vi "Import data from S2DS- B Reader.vi"(8 "error in (no error)":errorcluster) -> (0 "error out":errorcluster, 2 "Data out":dbl[](array[numeric]), 3 "connection out":refnum<k13>)   [LabVIEW 2016]
doc: "Uses DataSocket to read array data. \n \nThe Writer, Server, and Reader can all be on the same computer or different computers. The Writer and Reader URLs should point to the computer where the DataSocket Server is."
uses:
  source/INST DRIVERS/DilutionFridge/MyTriton.lvlib
panel:
  out "VISA resource name out":refnum<visa-resource-name>
  out "B":dbl
  in  "error in (no error) 2":errorcluster
  in  "VISA resource name in":refnum<visa-resource-name>="TCPIP0::192.168.0.107::33576::SOCKET"
  out "error out 2":errorcluster
  # "Overview: Demonstrates the use of the DataSocket functions to read data from the DataSocket server of S2DS.\nRequirements: Windows\nInstructions:\n1. Ensure Simple 2D Sweep : Export data  is TRUE.\n2. Run the VI."
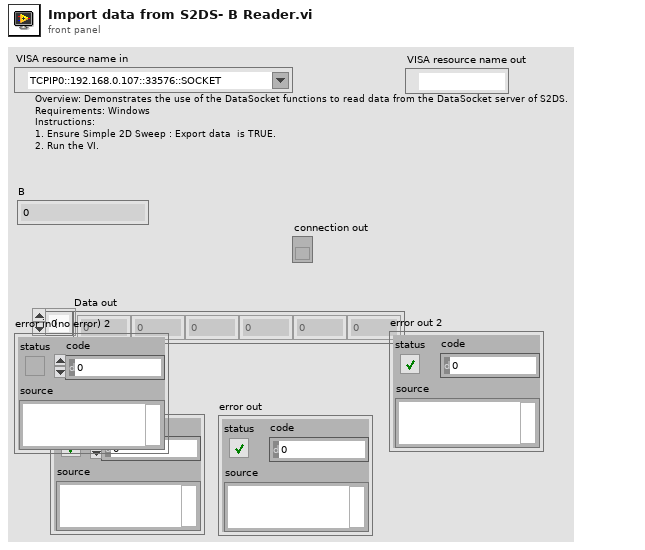
[diagram p1: front panel]
types:
  T1 = enum16{"Read", "Write", "ReadWrite", "BufferedRead", "BufferedReadWrite"}
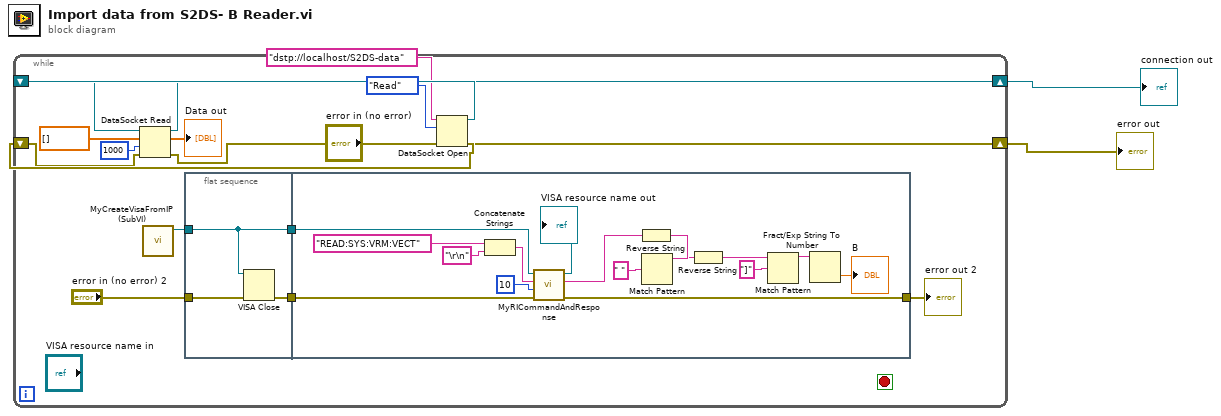
[diagram p0: block diagram]
diagram:
  n1 = DataSocket Open(8:"error in (no error)", 10:T1."Read" ("mode"), 11:"dstp://localhost/S2DS-data" ("Read Location")) -> (0:w4:errorcluster, 3:w6:refnum<k13>)  [unwired: 1 in]
  n2 = while {
    shift-right: [w13] -> w3
    shift-left: w6 -> [w15]
    shift-right: [w16] -> w7
    shift-left: w4 -> [w14]
    stop <- _ stop-if-true
    n3 = DataSocket Read(8:w14, 9:1000 ("ms timeout (10000)"), 10:dbl[] [], 11:w15) -> (0:w16:errorcluster, 2:→"Data out":dbl[], 3:w13:refnum<k13>)  [unwired: 5 out]
    n4 = call "MyCreateVisaFromIP (SubVI).vi"() -> ("VISA Refnum out"=w8:refnum<visa-resource-name>)  [unwired: 11 in]
    n5 = flat-sequence {
      tunnel: w8 -> [w20]
      tunnel: "error in (no error) 2" -> [w22]
      tunnel: [w21] -> w12
      tunnel: [w20] -> w11
      tunnel: w12 -> [w25]
      tunnel: w11 -> [w24]
      tunnel: [w23] -> w10
      frame #0 {
        n6 = VISA Close(VISA resource name=w20, error in (no error)=w22) -> (error out=w21:errorcluster)
      }
      frame #1 {
        n7 = Concatenate Strings("READ:SYS:VRM:VECT" ("Command"), "\r\n" ("string")) -> (w36:string)
        n8 = call "MyRICommandAndResponse.vi"("error in (no error)"=w25, "Min byte count"=u32 10 ("byte count"), "Command"=w36, "VISA resource name in"=w24) -> ("error out"=w23:errorcluster, "Response"=w30:string, "VISA resource name out"=→"VISA resource name out":refnum<visa-resource-name>)  [unwired: 5 in]
        n9 = Reverse String(1:w30) -> (0:w33:string)
        n10 = Match Pattern(string=w33, regular expression=" ") -> (before substring=w31:string)  [unwired: 1 in, 3 out]
        n11 = Reverse String(1:w31) -> (0:w29:string)
        n12 = Match Pattern(string=w29, regular expression="]") -> (before substring=w27:string)  [unwired: 1 in, 3 out]
        n13 = Fract/Exp String To Number(string=w27) -> (number=→"B":dbl)  [unwired: 3 in, 1 out]
      }
    }
    "error out 2" <- w10
  }
  "error out" <- w7
  "connection out" <- w3
